vi "array.vi"() -> ()   [LabVIEW 2014]
uses:
  <vilib>/myRIO/Common/Instrument Driver Framework/myRIO v1.0/UART/vis/myRIO v1.0 Close UART.vi
  <vilib>/myRIO/Common/Instrument Driver Framework/Utilities/vis/FPGA Ref Manager.vi
  <vilib>/myRIO/Common/Instrument Driver Framework/myRIO v1.0/myRIO v1.0 Reset FPGA.vi
  <vilib>/myRIO/Common/Instrument Driver Framework/myRIO v1.0/IRQ/vis/myRIO v1.0 IRQ Info FGV.vi
  <vilib>/myRIO/Common/Instrument Driver Framework/myRIO v1.0/IRQ/vis/myRIO v1.0 Timer IRQ Info FGV.vi
  <vilib>/myRIO/Common/Instrument Driver Framework/myRIO v1.0/IRQ/vis/myRIO v1.0 ISR Agent.vi
  <vilib>/myRIO/Instrument Drivers/Utilities/Utilities.lvlib
panel:
  in  "停止":bool
  out "Image":T1(plugin-control)
  out "Pixels Values":u8[][](array[numeric])
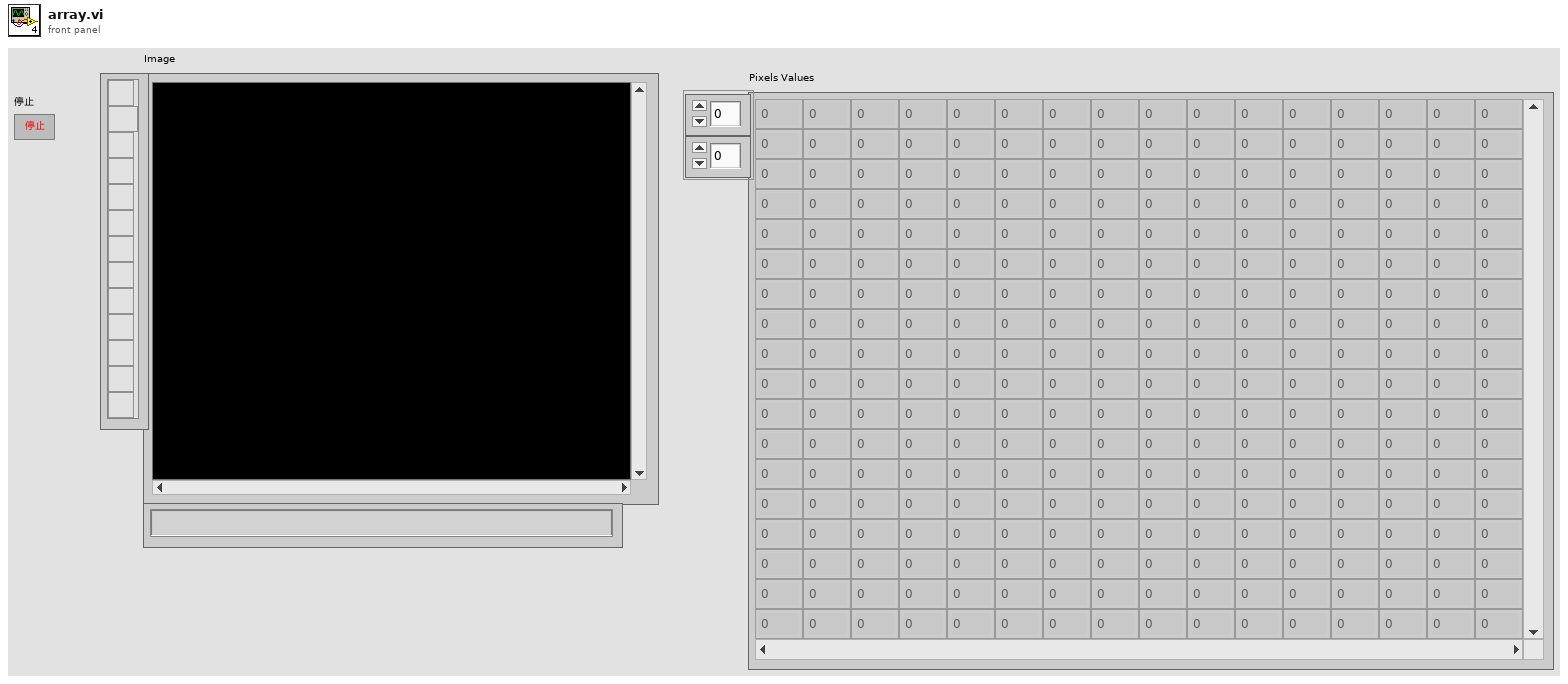
[diagram p1: front panel]
types:
  T1 = typedef "IMAQ Image.ctl" = refnum<image>
  T2 = cluster{"Optional Rectangle[0]":i32, "Optional Rectangle[1]":i32, "Optional Rectangle[2]":i32, "Optional Rectangle[3]":i32, "Optional Rectangle[4]":i32}
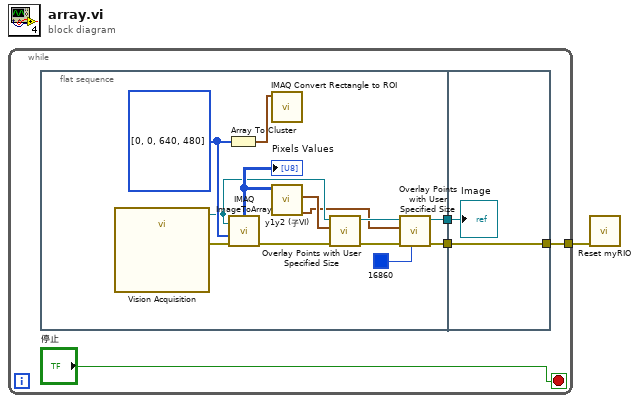
[diagram p0: block diagram]
diagram:
  n1 = while {
    tunnel: [w3] -> w1
    stop <- "停止" stop-if-true
    n2 = flat-sequence {
      tunnel: [w8] -> w5
      tunnel: [w9] -> w2
      tunnel: w5 -> [w20]
      tunnel: [w19] -> w3
      tunnel: w2 -> [w19]
      frame #0 {
        w16 = i32[] [0, 0, 640, 480] ("Optional Rectangle")
        n3 = call "Vision Acquisition"() -> ("Image Out"=w14:T1, "error out"=w13:errorcluster)  [unwired: 26 in]
        n4 = Array To Cluster(array=w16) -> (cluster=w18:T2)
        n5 = call "IMAQ ImageToArray"("error in (no error)"=w13, "Optional Rectangle"=w16, "Image"=w14) -> ("error out"=w12:errorcluster, "Image Pixels (U8)"=w17:u8[][])  [unwired: 1 in, 3 out]
        "Pixels Values" <- w17
        n6 = call "IMAQ Convert Rectangle to ROI"("Rectangle"=w18) -> ()  [unwired: 8 in, 2 out]
        n7 = call "y1y2 (子VI).vi"("Image Pixels (U8)输入"=w17) -> ("输出数组 2"=w7:cluster{i32, i32}[], "输出数组"=w15:cluster{i32, i32}[])  [unwired: 9 in]
        n8 = call "Overlay Points with User Specified Size.vi"("error in"=w12, "Points"=w15, "Image In"=w14) -> ("error out"=w11:errorcluster, "Image Out"=w10:T1)  [unwired: 7 in]
        n9 = call "Overlay Points with User Specified Size.vi"("Color"=u32 16860, "error in"=w11, "Points"=w7, "Image In"=w10) -> ("error out"=w9:errorcluster, "Image Out"=w8:T1)  [unwired: 6 in]
      }
      frame #1 {
        "Image" <- w20
      }
    }
  }
  n10 = call <vilib>:"Reset myRIO.vi"("error in (no error)"=w1) -> ()  [unwired: 10 in, 1 out]
